vi "Voltage Write Single.vi"(8 "error in":errorcluster, 9 "Channel Index":i32=1, 10 "Voltage.chX.AV":dbl, 11 "Device in":refnum<class "Device.lvclass">) -> (0 "error out":errorcluster, 3 "Device out":refnum<class "Device.lvclass">)   [LabVIEW 2023, in "Device.lvclass"]
uses:
  Device.lvclass
  Device.lvclass/Device.ctl
  Low Level Capabilities/Voltage/Voltage Actual Value/Voltage Actual Value.lvclass
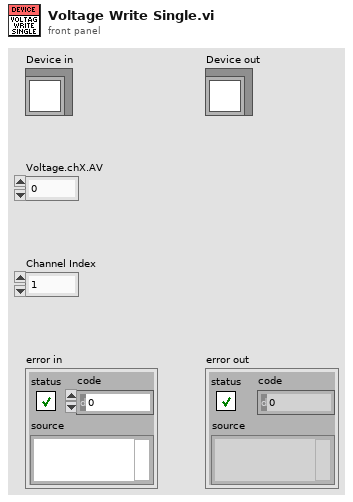
[diagram p1: front panel]
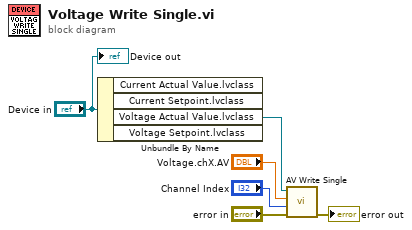
[diagram p0: block diagram]
diagram:
  n1 = Unbundle By Name("Device in") -> ("Voltage Actual Value.lvclass"=w4:refnum<class "Voltage Actual Value.lvclass">)  [unwired: 3 out]
  n2 = call-dynamic "AV Write Single.vi"("error in"="error in", "Channel Index"="Channel Index", "Voltage AV"="Voltage.chX.AV", "Voltage Actual Value in"=w4) -> ("error out"=→"error out":errorcluster)  [unwired: 6 in, 1 out]
  "Device out" <- "Device in"
